vi "ReadValveParameters.vi"   [LabVIEW 2014]
uses:
  axxon_Gold.vi
  <vilib>/Utility/file.llb/Read From Spreadsheet File (DBL).vi
types:
  T1 = cluster{"InitShutOff Distance：":dbl, "InitValve On Time：":dbl, "InitStay Time：":dbl, "InitValve On Delay：":dbl, "InitValve Pre-On Time：":dbl, "InitPre-Spray Time：":dbl, "InitSpeed：":dbl, "InitDispense Gap：":dbl, "InitPull Back Distance：":dbl, "InitStart Distance：":dbl, "InitEnd Distance:":dbl, "IinitLine":dbl, "Delaying spray off":dbl}
  T2 = cluster{"ShutOff Distance":dbl, "Valve On Time":dbl, "Stay Time":dbl, "Valve On Delay":dbl, "Valve Pre-On Time":dbl, "Pre-Spray Time":dbl, "Speed":dbl, "Dispense Gap":dbl, "Pull Back ":dbl, "Start Distance":dbl, "End Distance":dbl, "Line Width":dbl, "Delaying spray off":dbl}
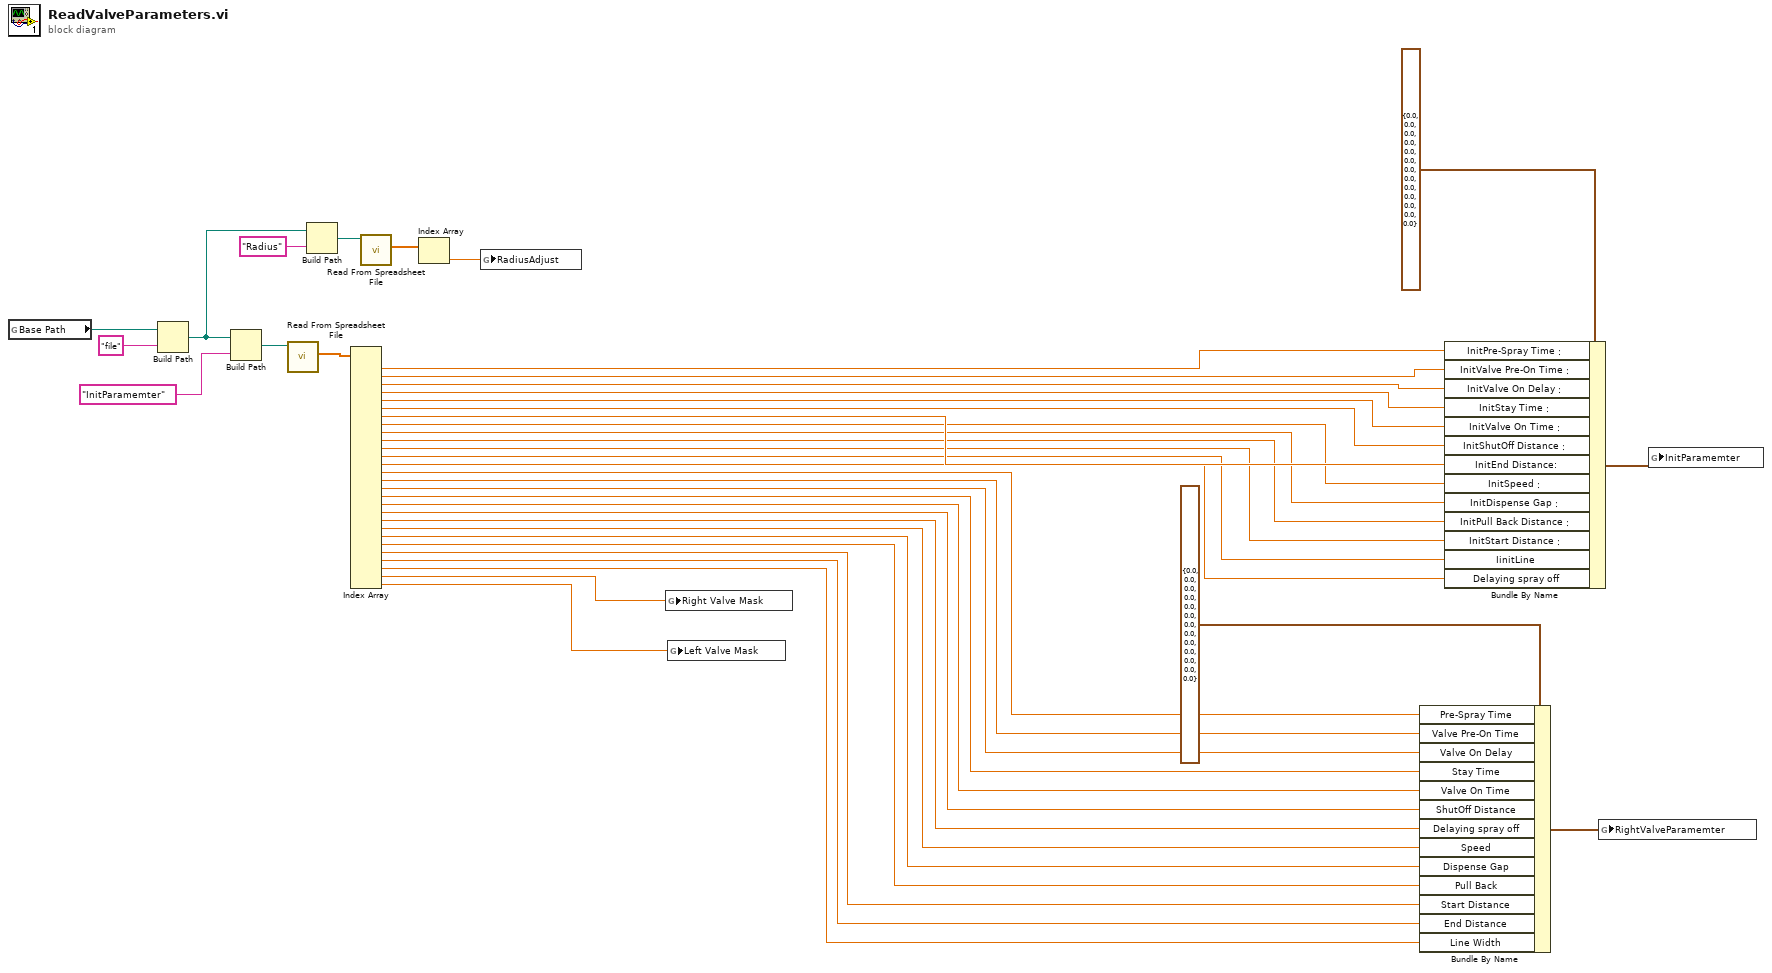
[diagram p0: block diagram]
diagram:
  n1 = global read "axxon_Gold.vi" "Base Path"() -> (w38:path)
  n2 = Build Path(base path=w38, name or relative path="file" ("名称或相对路径")) -> (appended path=w21:path)
  n3 = Build Path(base path=w21, name or relative path="InitParamemter" ("名称或相对路径")) -> (appended path=w41:path)
  n4 = call-poly <vilib>:"Read From Spreadsheet File.vi"("file path (dialog if empty)"=w41) -> ("first row"=w37:dbl[])  [unwired: 6 in, 4 out]
  n5 = Build Path(base path=w21, name or relative path="Radius" ("名称或相对路径")) -> (appended path=w24:path)
  n6 = Index Array(array=w37) -> (element #1=w36:dbl, element #2=w35:dbl, element #3=w34:dbl, element #4=w33:dbl, element #5=w32:dbl, element #6=w31:dbl, element #7=w30:dbl, element #8=w29:dbl, element #9=w28:dbl, element #10=w27:dbl, element #11=w26:dbl, element #12=w20:dbl, element #13=w1:dbl, element #14=w19:dbl, element #15=w18:dbl, element #16=w17:dbl, element #17=w16:dbl, element #18=w15:dbl, element #19=w14:dbl, element #20=w13:dbl, element #21=w12:dbl, element #22=w11:dbl, element #23=w10:dbl, element #24=w9:dbl, element #25=w8:dbl, element #26=w7:dbl, element #27=w6:dbl, element #28=w5:dbl)  [unwired: 28 in]
  n7 = call-poly <vilib>:"Read From Spreadsheet File.vi"("file path (dialog if empty)"=w24) -> ("first row"=w23:dbl[])  [unwired: 6 in, 4 out]
  n8 = Index Array(array=w23) -> (element=w22:dbl)  [unwired: 1 in]
  n9 = global write "axxon_Gold.vi" "RadiusAdjust"(w22) -> ()
  n10 = global write "axxon_Gold.vi" "Right Valve Mask"(w6) -> ()
  n11 = global write "axxon_Gold.vi" "Left Valve Mask"(w5) -> ()
  n12 = Bundle By Name(cluster=T2 {"ShutOff Distance"=0.0, "Valve On Time"=0.0, "Stay Time"=0.0, "Valve On Delay"=0.0, "Valve Pre-On Time"=0.0, "Pre-Spray Time"=0.0, "Speed"=0.0, "Dispense Gap"=0.0, "Pull Back "=0.0, "Start Distance"=0.0, "End Distance"=0.0, "Line Width"=0.0, "Delaying spray off"=0.0} ("RightValveParamemter"), "Pre-Spray Time"=w19, "Valve Pre-On Time"=w18, "Valve On Delay"=w17, "Stay Time"=w16, "Valve On Time"=w15, "ShutOff Distance"=w14, "Delaying spray off"=w13, "Speed"=w12, "Dispense Gap"=w11, "Pull Back"=w10, "Start Distance"=w9, "End Distance"=w8, "Line Width"=w7) -> (w4:T2)
  n13 = Bundle By Name(cluster=T1 {"InitShutOff Distance："=0.0, "InitValve On Time："=0.0, "InitStay Time："=0.0, "InitValve On Delay："=0.0, "InitValve Pre-On Time："=0.0, "InitPre-Spray Time："=0.0, "InitSpeed："=0.0, "InitDispense Gap："=0.0, "InitPull Back Distance："=0.0, "InitStart Distance："=0.0, "InitEnd Distance:"=0.0, "IinitLine"=0.0, "Delaying spray off"=0.0} ("InitParamemter"), "InitPre-Spray Time："=w36, "InitValve Pre-On Time："=w35, "InitValve On Delay："=w34, "InitStay Time："=w33, "InitValve On Time："=w32, "InitShutOff Distance："=w31, "InitEnd Distance:"=w30, "InitSpeed："=w29, "InitDispense Gap："=w28, "InitPull Back Distance："=w27, "InitStart Distance："=w26, "IinitLine"=w20, "Delaying spray off"=w1) -> (w42:T1)
  n14 = global write "axxon_Gold.vi" "RightValveParamemter"(w4) -> ()
  n15 = global write "axxon_Gold.vi" "InitParamemter"(w42) -> ()
